vi "Logg.vi"(3 "Pass":string, 4 "Datos":string, 5 "User":string) -> (0 "Logg":bool, 1 "Usuario":string, 2 "Usuarios":string[][](array[string]))   [LabVIEW 2017]
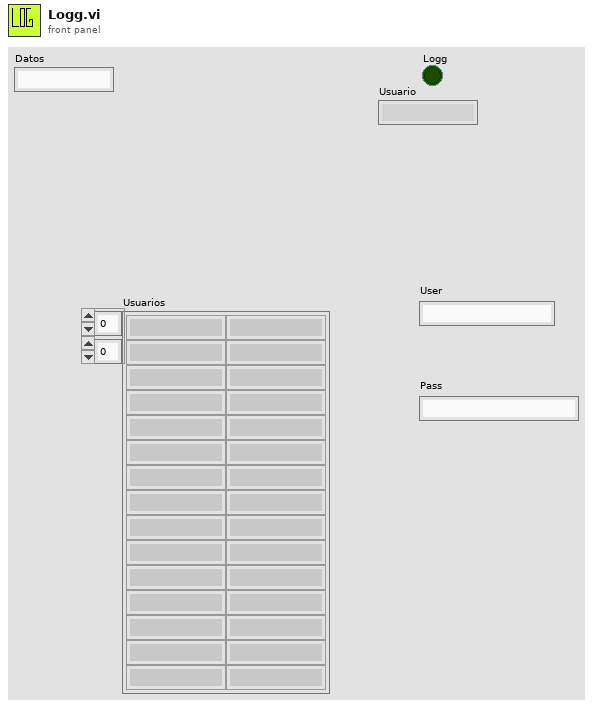
[diagram p1: front panel]
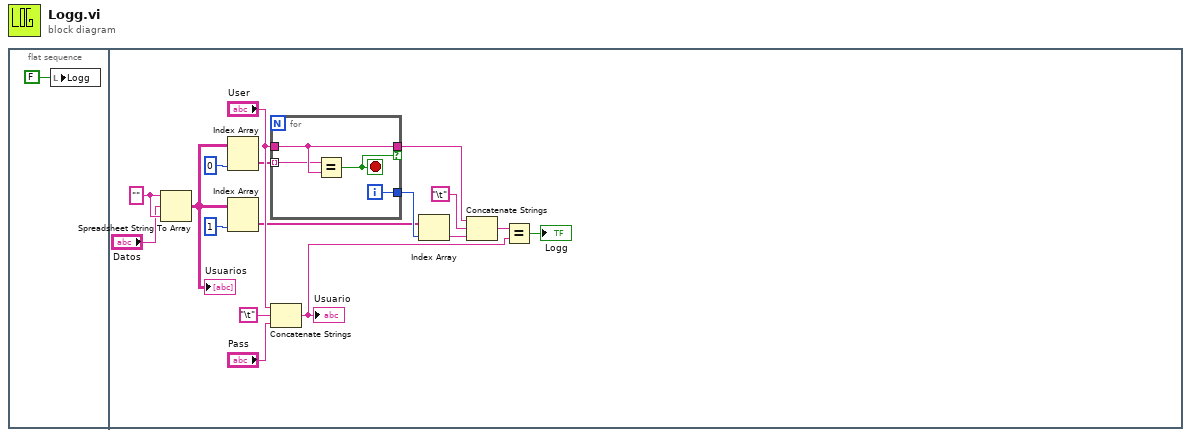
[diagram p0: block diagram]
diagram:
  n1 = flat-sequence {
    frame #0 {
      n2 = local write "Logg"(FALSE ("Logg")) -> ()
    }
    frame #1 {
      w17 = "" ("format string")
      n3 = Spreadsheet String To Array(format string=w17, spreadsheet string="Datos", array type (2D Dbl)=w17) -> (array=w6:string[][])  [unwired: 1 in]
      "Usuarios" <- w6
      n4 = Index Array(array=w6, index (col)=0 ("disabled index (col)")) -> (element=w7:string[])  [unwired: 1 in]
      n5 = Index Array(array=w6, index (col)=1 ("disabled index (col)")) -> (element=w3:string[])  [unwired: 1 in]
      n6 = for {
        tunnel: w7 -> [w19] mode=indexing
        tunnel: "User" -> [w22]
        tunnel: [w22] -> w14 if=w21
        tunnel: [w20] -> w4
        i -> [w20]
        stop <- w21 stop-if-true
        n7 = Equal?(x=w19, y=w22) -> (x = y?=w21:bool)
      }
      n8 = Concatenate Strings("User", "\t", "Pass") -> (w11:string)
      "Usuario" <- w11
      n9 = Index Array(array=w3, index=w4) -> (element=w2:string)
      n10 = Concatenate Strings(w14, "\t", w2) -> (w12:string)
      n11 = Equal?(x=w12, y=w11) -> (x = y?=→"Logg":bool)
    }
  }
